vi "Get Serializer.vi"(8 "error in (no error)":errorcluster, 11 "Record in":refnum<class "Record.lvclass">) -> (0 "error out":errorcluster, 2 "Serializer":refnum<class "Serializer.lvclass">, 3 "Record out":refnum<class "Record.lvclass">)   [LabVIEW 2017, in "Error Log.lvlib" / "Record.lvclass"]
uses:
  Record.lvclass
  Serializer/Serializer.lvclass
  Record.lvclass/Record.ctl
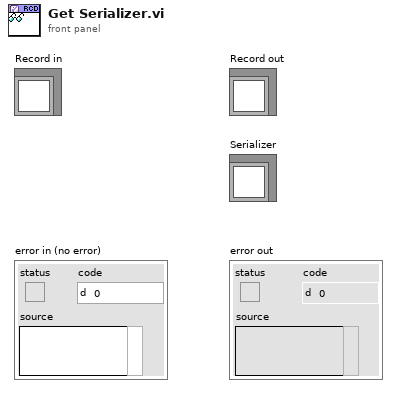
[diagram p1: front panel]
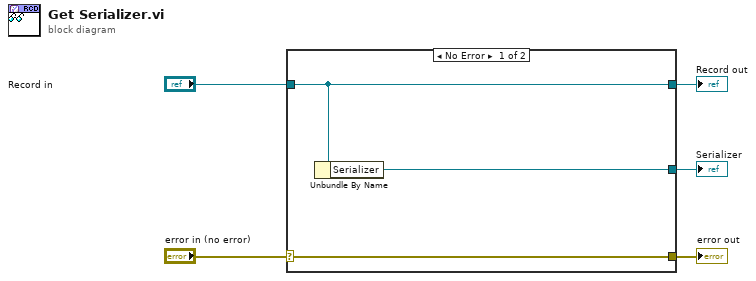
[diagram p0: block diagram]
diagram:
  n1 = case shown="No Error" "error in (no error)" {
    selector: "error in (no error)" -> [w8 w9]
    tunnel: [w8 w9] -> w4
    tunnel: [w7 w10] -> w2
    tunnel: "Record in" -> [w7 w10]
    tunnel: [w6 _] -> w1
    frame No Error {
      n2 = Unbundle By Name(w7) -> ("Serializer"=w6:refnum<class "Serializer.lvclass">)
    }
    frame Error {
    }
  }
  "error out" <- w4
  "Record out" <- w2
  "Serializer" <- w1
